vi "Get Command Handling.vi"(8 "error in (no error)":errorcluster) -> (0 "error out":errorcluster, 3 "Command Handling Disabled?":bool)   [LabVIEW 2015, in "Command Handler.lvlib"]
uses:
  Command Handler.lvlib
  Command Handler Global.vi
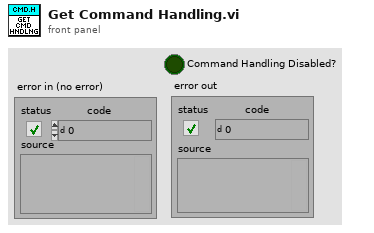
[diagram p1: front panel]
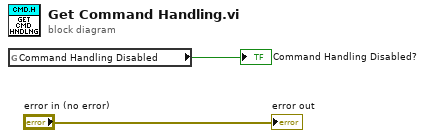
[diagram p0: block diagram]
diagram:
  n1 = global read "Command Handler Global.vi" "Command Handling Disabled"() -> (→"Command Handling Disabled?":bool)
  "error out" <- "error in (no error)"
